vi "SP Check Segmented Limit (array X Y).vi"(0 "Specification Cluster":cluster{"X":dbl[], "Y":dbl[]}[](array[cluster]) {"Y" format="%0.2f"; "X" format="%0.2f"}, 1 "x0":dbl format="%0.2f", 2 "dx":dbl format="%0.2f", 3 "error in":errorcluster) -> (8 "limit spec ok":bool, 9 "1st valid segment index":i32, 10 "error out":errorcluster)   [LabVIEW 2011]
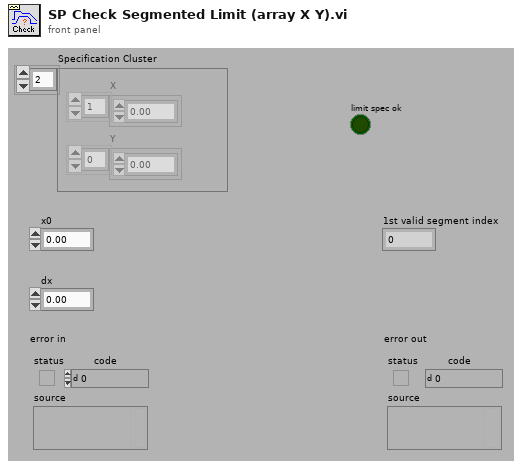
[diagram p1: front panel]
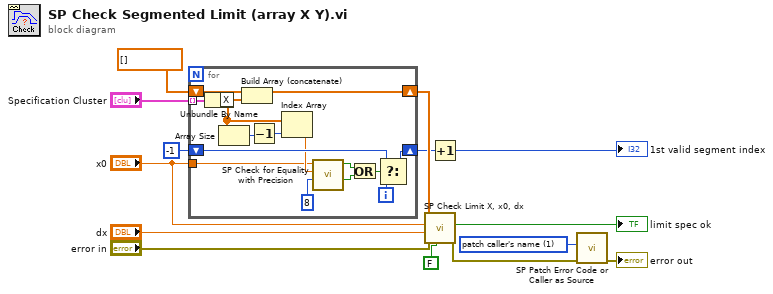
[diagram p0: block diagram]
diagram:
  w4 = u16 1 items=["patch error code", "patch caller's name"] ("operation")
  n1 = for {
    tunnel: "Specification Cluster" -> [w29] mode=indexing
    shift-right: [w15] -> w10
    shift-left: dbl[] [] ("element") -> [w28]
    shift-right: [w24] -> w6
    shift-left: -1 -> [w25]
    tunnel: "x0" -> [w20]
    i -> [w22]
    n2 = Unbundle By Name(w29) -> ("X"=w23:dbl[])
    n3 = Array Size(array=w23) -> (size(s)=w27:i32)
    n4 = Build Array (concatenate)(w28, w23) -> (w15:dbl[])
    n5 = Decrement(x=w27) -> (x-1=w26:i32)
    n6 = Index Array(array=w23, index=w26) -> (element=w21:dbl)
    n7 = call "SP Check for Equality with Precision.vi"("precision"=8, "n2"=w21, "n1"=w20) -> ("n1 < n2?"=w17:bool, "equal (within precision)"=w18:bool)  [unwired: 7 out]
    n8 = Or(x=w18, y=w17) -> (x .or. y?=w16:bool)
    n9 = Select(t=w25, s=w16, f=w22) -> (s? t:f=w24:i32)
  }
  n10 = call "SP Check Limit X, x0, dx.vi"("X"=w10, "x0"="x0", "dX"="dx", "error in"="error in", "Check x0? (T)"=FALSE) -> ("Limit Spec OK"=→"limit spec ok":bool, "error out"=w3:errorcluster)  [unwired: 4 out]
  n11 = Increment(x=w6) -> (x+1=→"1st valid segment index":i32)
  n12 = call "SP Patch Error Code or Caller as Source.vi"("error in (no error)"=w3, "operation"=w4) -> ("error out"=→"error out":errorcluster)  [unwired: 2 in, 7 out]
